vi "First Step.vi"(8 "error in (no error)":errorcluster, 11 "Pulse Gen Basic Scan.lvclass in":refnum<class "Pulse Gen Basic Scan.lvclass">) -> (0 "error out":errorcluster, 2 "Current Position":dbl, 3 "Pulse Gen Basic Scan.lvclass out":refnum<class "Pulse Gen Basic Scan.lvclass">)   [LabVIEW 2009, in "Pulse Gen Basic Scan.lvclass"]
doc: "(Dynamic) Reset the instrument and prepare to scan. Go to step #0 - the first step. If desired, the scanner may do this in a different way than usual (i.e. by preparing to move a long distance, or reset to home position.)"
uses:
  Pulse Gen Basic Scan.lvclass
  Scanner/Scanner.lvclass
  Instruments/Utility Classes/Scannable/Scannable.lvclass
  Pulse Gen Basic Scan.lvclass/Pulse Gen Basic Scan.ctl
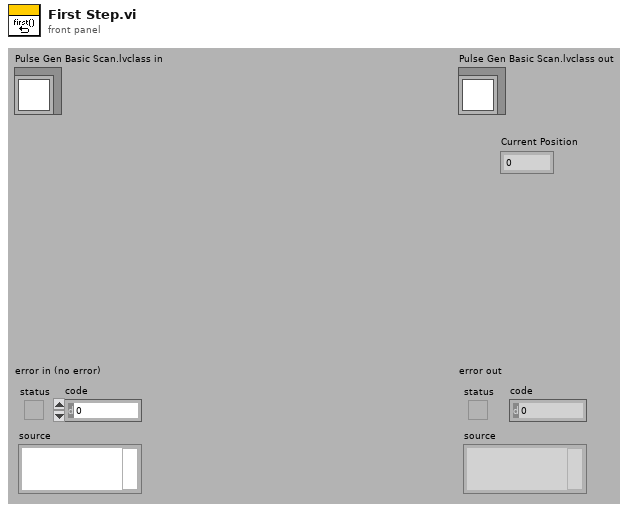
[diagram p1: front panel]
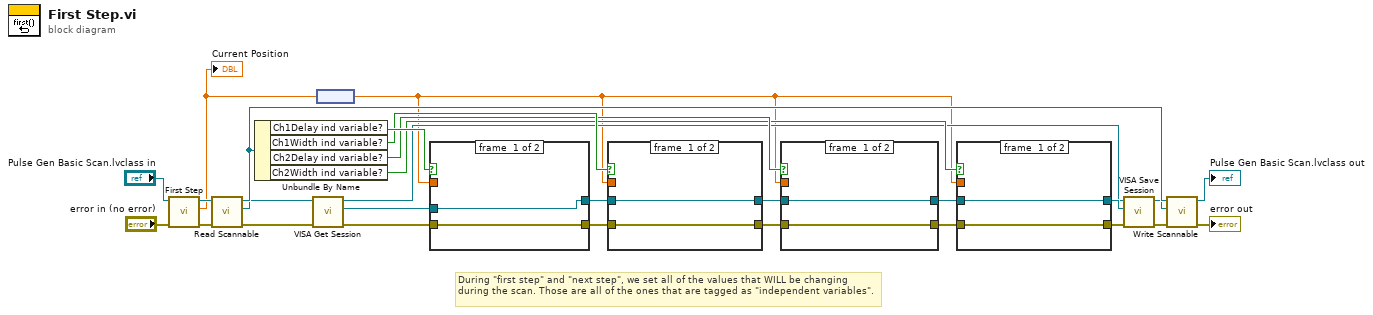
[diagram p0: block diagram]
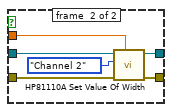
[diagram p2: hidden frame]
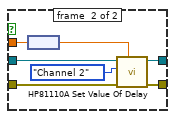
[diagram p3: hidden frame]
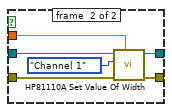
[diagram p4: hidden frame]
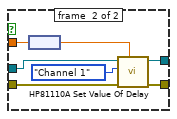
[diagram p5: hidden frame]
diagram:
  # "During \"first step\" and \"next step\", we set all of the values that WILL be changing during the scan. Those are all of the ones that are tagged as \"independent variables\"."
  n1 = call-parent "First Step.vi"("error in (no error)"="error in (no error)", "Scanner.lvclass in"="Pulse Gen Basic Scan.lvclass in") -> ("error out"=w13:errorcluster, "Current Position"=w3:dbl, "Scanner.lvclass out"=w16:refnum<class "Pulse Gen Basic Scan.lvclass">)  [unwired: 7 in]
  "Current Position" <- w3
  n2 = call-dynamic "Read Scannable.vi"("error in (no error)"=w13, "Scanner.lvclass in"=w16) -> ("error out"=w12:errorcluster, "Scannable.lvclass"=w9:refnum<class "Scannable.lvclass">, "Scanner.lvclass out"=w15:refnum<class "Pulse Gen Basic Scan.lvclass">)  [unwired: 7 out]
  n3 = Unbundle By Name(w15) -> ("Ch1Delay ind variable?"=w20:bool, "Ch1Width ind variable?"=w19:bool, "Ch2Delay ind variable?"=w18:bool, "Ch2Width ind variable?"=w17:bool)
  n4 = call-dynamic "VISA Get Session.vi"("error in (no error)"=w12, "Instrument.lvclass in"=w9) -> ("error out"=w11:errorcluster, "VISA Resource Name"=w1:refnum<visa-resource-name>, "Instrument.lvclass out"=w8:refnum<class "Scannable.lvclass">)  [unwired: 7 out]
  n5 = node(w3) -> (w2:dbl[unit])
  n6 = case shown="True" w20 {
    tunnel: [w29 w37] -> w26
    tunnel: w11 -> [w30 w36]
    tunnel: [w30 w35] -> w23
    tunnel: w2 -> [_ w33]
    tunnel: w1 -> [w29 w31]
    frame #0 {
    }
    frame #1 {
      n7 = node(w33) -> (w32:dbl)
      n8 = call "HP81110A Set Value Of Delay.vi"("Delay Value (0.0)"=w32, "error in (no error)"=w36, "Channel (1:Channel 1)"=enum16{"Channel All ", "Channel 1", "Channel 2"}."Channel 1", "VISA session"=w31) -> ("error out"=w35:errorcluster, "dup VISA session"=w37:refnum<visa-resource-name>)  [unwired: 6 in]
    }
  }
  n9 = case shown="True" w19 {
    tunnel: w26 -> [w39 w45]
    tunnel: [w39 w44] -> w25
    tunnel: w23 -> [w38 w43]
    tunnel: [w38 w42] -> w22
    tunnel: w2 -> [_ w40]
    frame #0 {
    }
    frame #1 {
      n10 = call "HP81110A Set Value Of Width.vi"("Width Value (100.0E-9)"=w40, "error in (no error)"=w43, "Channel (1:Channel 1)"=enum16{"Channel All ", "Channel 1", "Channel 2"}."Channel 1", "VISA session"=w45) -> ("error out"=w42:errorcluster, "dup VISA session"=w44:refnum<visa-resource-name>)  [unwired: 6 in]
    }
  }
  n11 = case shown="True" w18 {
    tunnel: w25 -> [w47 w54]
    tunnel: [w47 w53] -> w24
    tunnel: w22 -> [w46 w52]
    tunnel: [w46 w51] -> w21
    tunnel: w2 -> [_ w49]
    frame #0 {
    }
    frame #1 {
      n12 = node(w49) -> (w48:dbl)
      n13 = call "HP81110A Set Value Of Delay.vi"("Delay Value (0.0)"=w48, "error in (no error)"=w52, "Channel (1:Channel 1)"=enum16{"Channel All ", "Channel 1", "Channel 2"}."Channel 2", "VISA session"=w54) -> ("error out"=w51:errorcluster, "dup VISA session"=w53:refnum<visa-resource-name>)  [unwired: 6 in]
    }
  }
  n14 = case shown="True" w17 {
    tunnel: w24 -> [w55 w62]
    tunnel: w21 -> [w56 w61]
    tunnel: [w56 w60] -> w6
    tunnel: w2 -> [_ w58]
    tunnel: [w55 w57] -> w10
    frame #0 {
    }
    frame #1 {
      n15 = call "HP81110A Set Value Of Width.vi"("Width Value (100.0E-9)"=w58, "error in (no error)"=w61, "Channel (1:Channel 1)"=enum16{"Channel All ", "Channel 1", "Channel 2"}."Channel 2", "VISA session"=w62) -> ("error out"=w60:errorcluster, "dup VISA session"=w57:refnum<visa-resource-name>)  [unwired: 6 in]
    }
  }
  n16 = call-dynamic "VISA Save Session.vi"("error in (no error)"=w6, "VISA Resource Name"=w10, "Instrument.lvclass in"=w8) -> ("error out"=w5:errorcluster, "Instrument.lvclass out"=w7:refnum<class "Scannable.lvclass">)  [unwired: 7 out]
  n17 = call-dynamic "Write Scannable.vi"("error in (no error)"=w5, "Scannable.lvclass"=w7, "Scanner.lvclass in"=w15) -> ("error out"=→"error out":errorcluster, "Scanner.lvclass out"=→"Pulse Gen Basic Scan.lvclass out":refnum<class "Pulse Gen Basic Scan.lvclass">)  [unwired: 7 out]
